vi "Perform Action.vi"(8 "error in (no error)":errorcluster, 10 "Input":variant, 11 "DIO DAQmx PWM CFG in":refnum<class "CO DAQmx PWM CFG.lvclass">) -> (0 "error out":errorcluster, 2 "Output":variant, 3 "DIO DAQmx PWM CFG out":refnum<class "CO DAQmx PWM CFG.lvclass">)   [LabVIEW 2023, in "DAQmx Simulated CFGs.lvlib" / "CO DAQmx PWM CFG.lvclass"]
uses:
  CO DAQmx PWM CFG.lvclass
  CO DAQmx PWM CFG/CO DAQmx PWM CFG.lvclass
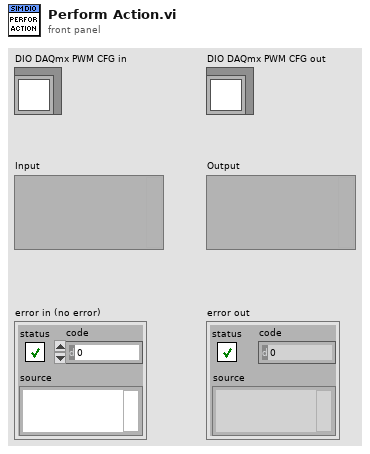
[diagram p1: front panel]
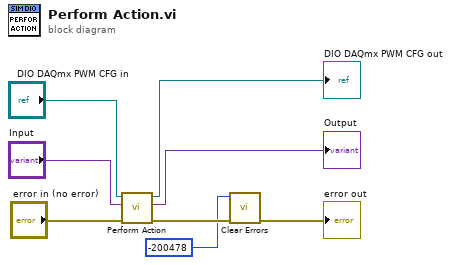
[diagram p0: block diagram]
diagram:
  n1 = call-parent "Perform Action.vi"("error in (no error)"="error in (no error)", "Input"="Input", "DIO DAQmx PWM CFG in"="DIO DAQmx PWM CFG in") -> ("error out"=w8:errorcluster, "Output"=→"Output":variant, "DIO DAQmx PWM CFG out"=→"DIO DAQmx PWM CFG out":refnum<class "CO DAQmx PWM CFG.lvclass">)  [unwired: 6 in]
  n2 = call <vilib>:"Clear Errors.vi"("error in (no error)"=w8, "specific error code to clear (0: all)"=-200478) -> ("error out"=→"error out":errorcluster)  [unwired: 4 in, 1 out]
